vi "VariableOfScript.vi"(8 "error in (no error)":errorcluster, 10 "Cluster":T1={"MZ Start"=15000.0, "MZ End"=100000.0, "MZ Target"=25000.0, "Laser Shots"=3.0, "MZ Aux Scan Start"=25000.0, "MZ Aux Scan Stop"=40000.0, "Aux Amp"=1.0}, 11 "RawScripeString":string) -> (0 "error out":errorcluster, 3 "RawScripeString Output":string)   [LabVIEW 2018]
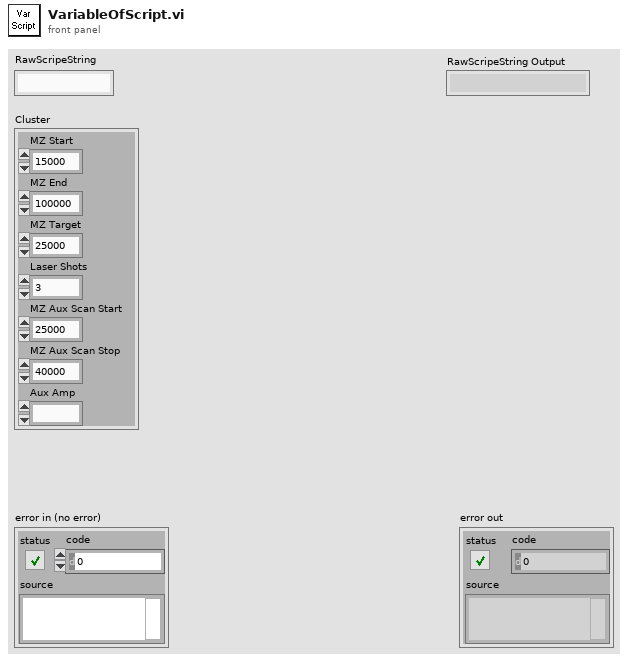
[diagram p1: front panel]
types:
  T1 = cluster{"MZ Start":dbl, "MZ End":dbl, "MZ Target":dbl, "Laser Shots":dbl, "MZ Aux Scan Start":dbl, "MZ Aux Scan Stop":dbl, "Aux Amp":ext}
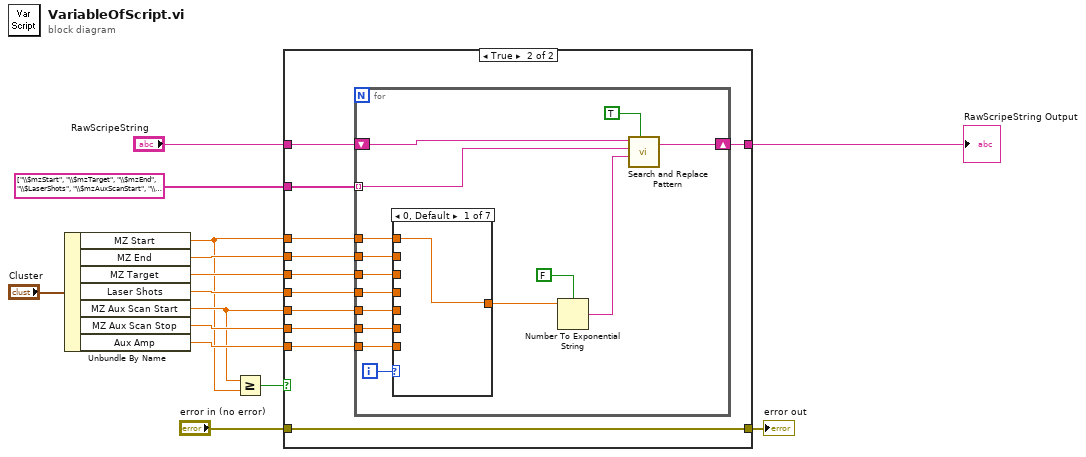
[diagram p0: block diagram]
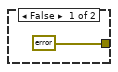
[diagram p2: hidden frame]
diagram:
  n1 = Unbundle By Name("Cluster") -> ("MZ Start"=w4:dbl, "MZ End"=w12:dbl, "MZ Target"=w11:dbl, "Laser Shots"=w10:dbl, "MZ Aux Scan Start"=w5:dbl, "MZ Aux Scan Stop"=w9:dbl, "Aux Amp"=w8:ext)
  n2 = Greater Or Equal?(x=w5, y=w4) -> (x >= y?=w3:bool)
  n3 = case shown="True" w3 {
    tunnel: string[] ["\\$mzStart", "\\$mzTarget", "\\$mzEnd", "\\$LaserShots", "\\$mzAuxScanStart", "\\$mzAuxScanStop", "\\$AuxAmp"] -> [_ w26]
    tunnel: w12 -> [_ w25]
    tunnel: w11 -> [_ w24]
    tunnel: w10 -> [_ w23]
    tunnel: w9 -> [_ w22]
    tunnel: w8 -> [_ w21]
    tunnel: "RawScripeString" -> [_ w20]
    tunnel: [_ w19] -> w6
    tunnel: w5 -> [_ w18]
    tunnel: w4 -> [_ w17]
    tunnel: "error in (no error)" -> [_ w16]
    tunnel: [errorcluster {"status"=TRUE, "code"=5666, "source"="Input Error"} ("error in (no error)") w16] -> w1
    frame False {
    }
    frame True {
      n4 = for {
        tunnel: w26 -> [w31] mode=indexing
        tunnel: w17 -> [w40]
        tunnel: w25 -> [w38]
        tunnel: w24 -> [w37]
        tunnel: w23 -> [w36]
        tunnel: w18 -> [w35]
        tunnel: w22 -> [w34]
        tunnel: w21 -> [w33]
        shift-right: [w28] -> w19
        shift-left: w20 -> [w32]
        i -> [w41]
        n5 = case shown="0, Default" w41 {
          tunnel: w40 -> [w42 _ _ _ _ _ _]
          tunnel: [w42 w43 w44 w45 w46 w47 w48] -> w39
          tunnel: w38 -> [_ w43 _ _ _ _ _]
          tunnel: w37 -> [_ _ w44 _ _ _ _]
          tunnel: w36 -> [_ _ _ w45 _ _ _]
          tunnel: w35 -> [_ _ _ _ w46 _ _]
          tunnel: w34 -> [_ _ _ _ _ w47 _]
          tunnel: w33 -> [_ _ _ _ _ _ w48]
          frame 0, Default {
          }
          frame 1 {
          }
          frame 2 {
          }
          frame 3 {
          }
          frame 4 {
          }
          frame 5 {
          }
          frame 6 {
          }
        }
        n6 = Number To Exponential String(number=w39, 1:FALSE ("use system decimal point (T)")) -> (E-format string=w30:string)  [unwired: 2 in]
        n7 = call <vilib>:"Search and Replace Pattern.vi"("string"=w32, "regular expression (\"\")"=w31, "replace string (\"\")"=w30, "replace all? (F)"=TRUE) -> ("result string"=w28:string)  [unwired: 1 in, 1 out]
      }
    }
  }
  "RawScripeString Output" <- w6
  "error out" <- w1
